vi "Multiple Register.vi"() -> ()   [LabVIEW 2024]
uses:
  Registry.lvlib
  Logger/Logger.lvclass
panel:
  out "multiple register test":bool
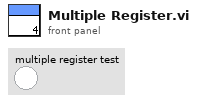
[diagram p1: front panel]
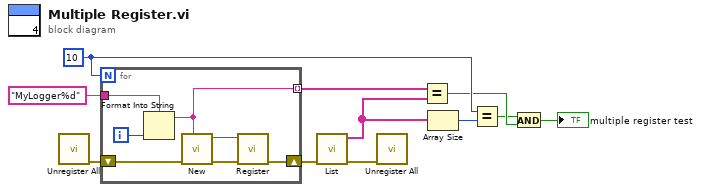
[diagram p0: block diagram]
diagram:
  w10 = 10
  n1 = call "Unregister All.vi"() -> ("error out"=w3:errorcluster)  [unwired: 10 in, 1 out]
  n2 = for {
    N: w10 -> [_]
    tunnel: "MyLogger%d" ("name") -> [w16]
    tunnel: [w15] -> w9 mode=indexing
    shift-right: [w12] -> w2
    shift-left: w3 -> [w14]
    i -> [w17]
    n3 = Format Into String(format string=w16, w17) -> (resulting string=w15:string)  [unwired: 2 in, 1 out]
    n4 = call "New.vi"("name (\"Default\")"=w15, "error in (no error)"=w14) -> ("error out"=w13:errorcluster, "logger"=w18:refnum<class "Logger.lvclass">)  [unwired: 8 in]
    n5 = call "Register.vi"("error in (no error)"=w13, "logger in"=w18) -> ("error out"=w12:errorcluster)  [unwired: 9 in]
  }
  n6 = call "List.vi"("error in (no error)"=w2) -> ("error out"=w1:errorcluster, "registered loggers"=w8:string[])  [unwired: 9 in]
  n7 = call "Unregister All.vi"("error in (no error)"=w1) -> ()  [unwired: 9 in, 2 out]
  n8 = Equal?(x=w9, y=w8) -> (x = y?=w7:bool)
  n9 = Array Size(array=w8) -> (size(s)=w11:i32)
  n10 = Equal?(x=w10, y=w11) -> (x = y?=w5:bool)
  n11 = And(x=w5, y=w7) -> (x .and. y?=→"multiple register test":bool)
